vi "是否处在运行状态.vi"   [LabVIEW 2011]
types:
  T1 = enum32{"Invalid", "Standard", "Closed", "Hidden", "Minimized", "Maximized"}
  T2 = enum32{"Bad", "Idle", "Run top level", "Running"}
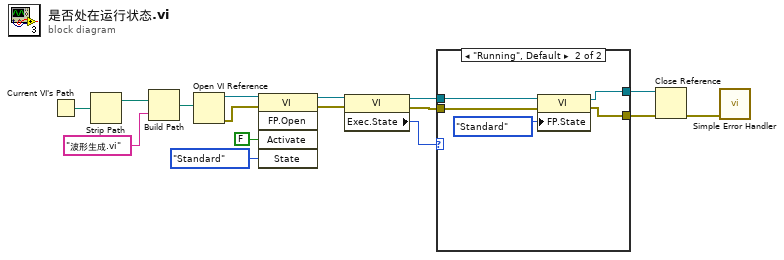
[diagram p0: block diagram]
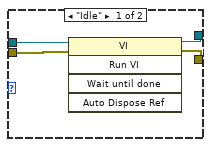
[diagram p2: hidden frame]
diagram:
  n1 = Current VI's Path() -> (path=w16:path)
  n2 = Strip Path(path=w16) -> (stripped path=w15:path)  [unwired: 1 out]
  n3 = Build Path(base path=w15, name or relative path="波形生成.vi") -> (appended path=w13:path)
  n4 = Open VI Reference(vi path=w13) -> (vi reference=w12:refnum<vi>, error out=w11:errorcluster)  [unwired: 5 in]
  n5 = invoke class="VI" method="FP.Open"(reference=w12, error in=w11, "Activate"=FALSE ("Activate?"), "State"=T1."Standard") -> (reference out=w8:refnum<vi>, error out=w7:errorcluster)  [unwired: 1 in, 3 out]
  n6 = property class="VI"(reference=w8, error in=w7) -> (reference out=w5:refnum<vi>, error out=w4:errorcluster, "Exec.State"=w6:T2)
  n7 = case shown="\"Running\", Default" w6 {
    tunnel: w5 -> [w20 w25]
    tunnel: w4 -> [w19 w24]
    tunnel: [w18 w23] -> w3
    tunnel: [w17 w22] -> w2
    frame "Idle" {
      n8 = invoke class="VI" method="Run VI"(reference=w20, error in=w19) -> (reference out=w18:refnum<vi>, error out=w17:errorcluster)  [unwired: 3 in, 3 out]
    }
    frame "Running", Default {
      n9 = property class="VI"(reference=w25, error in=w24, "FP.State"=T1."Standard" ("Front Panel Window:State")) -> (reference out=w23:refnum<vi>, error out=w22:errorcluster)
    }
  }
  n10 = Close Reference(reference=w3, error in (no error)=w2) -> (error out=w1:errorcluster)
  n11 = call <vilib>:"Simple Error Handler.vi"("error in (no error)"=w1) -> ()  [unwired: 4 in, 5 out]
